vi "getTempMov.vi"() -> ()   [LabVIEW 2017]
panel:
  in  "数据":dbl[](array[numeric])
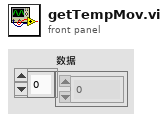
[diagram p1: front panel]
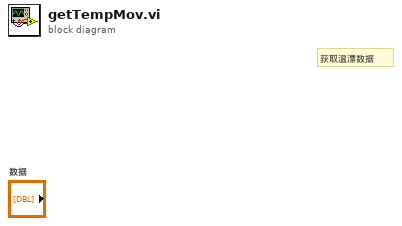
[diagram p0: block diagram]
diagram:
  # "获取温漂数据"
